vi "I-V to Waveform parameters.vi"(9 "Input range":dbl=1.0 format="%#_6p", 11 "I-V parameters":T1={"Start magnitude"=0.001, "Magnitude increment"=0.001, "End magnitude"=7.0, "Ramp length"=32, "Top  length"=480, "Threshold "=0.0001, "Processing delay"=255, "Valhalla range"=0.01, "Interpolation"=64, "Stop after"=1, "Detector window"=480} {"Detector window" format="%dpts"; "Stop after" format="%d sweep(s)"; "Valhalla range" format="%#_6pA"; "Processing delay" format="%dpts"; "Threshold" format="%#_6pV"; "Top  length" format="%dpts"; "Ramp length" format="%dpts"; "End magnitude" format="%#_6pA"; "Magnitude increment" format="%#_6pA"; "Start magnitude" format="%#_6pA"}) -> (3 "Waveform parameters out":T2={"Start magnitude"=1000.0, "Magnitude increment"=500.0, "Number of pulses"=8, "Ramp length"=32, "Top  length"=480, "Threshold "=15729, "Processing delay"=240, "Stop after"=1, "Detector window"=480} {"Detector window" format="%dpts"; "Stop after" format="%d sweep(s)"})   [LabVIEW 2019]
uses:
  Waveform parameters.ctl
  I-V parameters.ctl
panel:
  out "End In Range?":bool
  out "Start In Range?":bool
  # "Waveform parameters"
  # "Detector parameters"
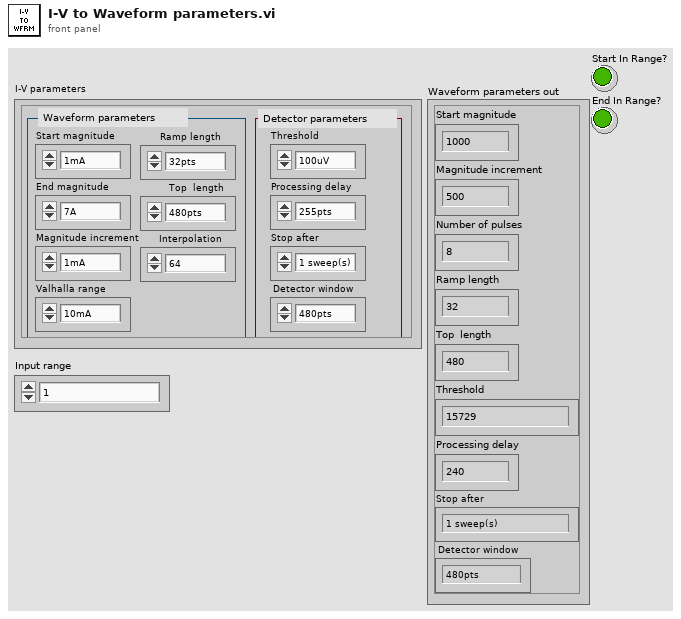
[diagram p1: front panel]
types:
  T1 = typedef "I-V parameters.ctl" = cluster{"Start magnitude":dbl, "Magnitude increment":dbl, "End magnitude":dbl, "Ramp length":i32, "Top  length":i32, "Threshold ":dbl, "Processing delay":u16, "Valhalla range":dbl, "Interpolation":i32, "Stop after":u16, "Detector window":i32}
  T2 = typedef "Waveform parameters.ctl" = cluster{"Start magnitude":dbl, "Magnitude increment":dbl, "Number of pulses":i32, "Ramp length":i32, "Top  length":i32, "Threshold ":i32, "Processing delay":u16, "Stop after":u16, "Detector window":i32}
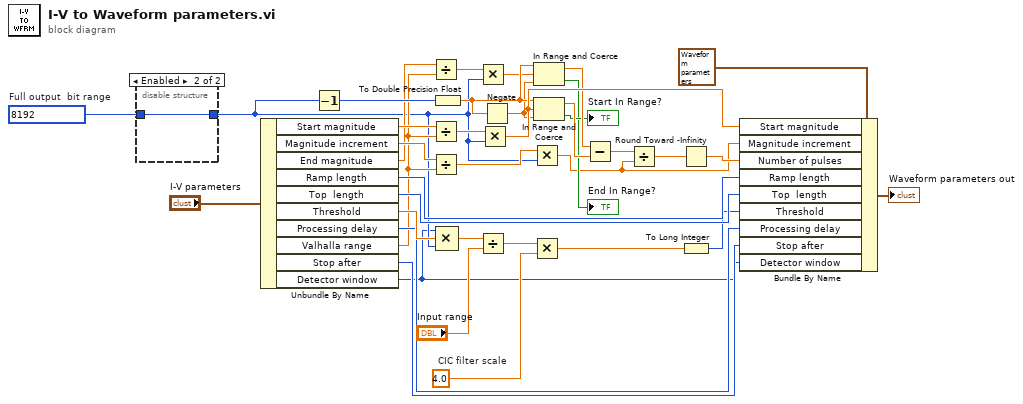
[diagram p0: block diagram]
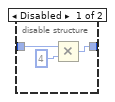
[diagram p2: hidden frame]
diagram:
  w22 = 4.0  # CIC filter scale
  w7 = 8192  # Full output  bit range
  n1 = disable-structure shown="Enabled" {
    disable-tunnel: w7 -> [w40 w41]
    disable-tunnel: [w39 w41] -> w3
    frame Disabled {
      n2 = Multiply(x=w40, y=4) -> (x*y=w39:i32)
    }
    frame Enabled {
    }
  }
  n3 = Unbundle By Name("I-V parameters") -> ("Start magnitude"=w21:dbl, "Magnitude increment"=w26:dbl, "End magnitude"=w17:dbl, "Ramp length"=w34:i32, "Top  length"=w33:i32, "Threshold"=w32:dbl, "Processing delay"=w28:u16, "Valhalla range"=w9:dbl, "Stop after"=w2:u16, "Detector window"=w1:i32)
  n4 = Decrement(x=w3) -> (x-1=w19:i32)
  n5 = Divide(x=w17, y=w9) -> (x/y=w10:dbl)
  n6 = Divide(x=w21, y=w9) -> (x/y=w25:dbl)
  n7 = Divide(x=w26, y=w9) -> (x/y=w27:dbl)
  n8 = To Double Precision Float(number=w19) -> (double precision float=w16:dbl)
  n9 = Compound Arithmetic op=MULTIPLY(w1, w32, w3) -> (w31:dbl)
  n10 = Multiply(x=w10, y=w3) -> (x*y=w8:dbl)
  n11 = Divide(x=w31, y="Input range") -> (x/y=w23:dbl)
  n12 = Multiply(x=w25, y=w3) -> (x*y=w18:dbl)
  n13 = Negate(x=w16) -> (-x=w15:dbl)
  n14 = Multiply(x=w27, y=w3) -> (x*y=w4:dbl)
  n15 = Multiply(x=w23, y=w22) -> (x*y=w24:dbl)
  n16 = In Range and Coerce(upper limit=w16, x=w8, lower limit=w15) -> (coerced(x)=w14:dbl, In Range?=→"End In Range?":bool)
  n17 = In Range and Coerce(upper limit=w16, x=w18, lower limit=w15) -> (coerced(x)=w13:dbl, In Range?=→"Start In Range?":bool)
  n18 = Subtract(x=w14, y=w13) -> (x-y=w5:dbl)
  n19 = Divide(x=w5, y=w4) -> (x/y=w6:dbl)
  n20 = Round Toward -Infinity(1:w6) -> (0:w20:dbl)
  n21 = To Long Integer(number=w24) -> (32bit integer=w29:i32)
  n22 = Bundle By Name(cluster=T2 {"Start magnitude"=1000.0, "Magnitude increment"=500.0, "Number of pulses"=8, "Ramp length"=32, "Top  length"=480, "Threshold "=3000, "Processing delay"=240, "Stop after"=1, "Detector window"=480} ("Waveform parameters out"), "Start magnitude"=w18, "Magnitude increment"=w4, "Number of pulses"=w20, "Ramp length"=w34, "Top  length"=w33, "Threshold"=w29, "Processing delay"=w28, "Stop after"=w2, "Detector window"=w1) -> (→"Waveform parameters out":T2)
